vi "Get Camera Configuration.vi"(8 "error in (no error)":errorcluster, 11 "NI Vision Camera in":refnum<class "NI Vision Camera.lvclass">) -> (0 "error out":errorcluster, 2 "Configuration":T1, 3 "NI Vision Camera out":refnum<class "NI Vision Camera.lvclass">)   [LabVIEW 2014, in "NI Vision Camera.lvclass"]
uses:
  NI Vision Camera.lvclass
  Configuration.ctl
  NI Vision Camera.lvclass/NI Vision Camera.ctl
  <resource>/objmgr/imaqdx.rc
  Framework/Interfaces/Observable Actor/Observable Actor.lvclass
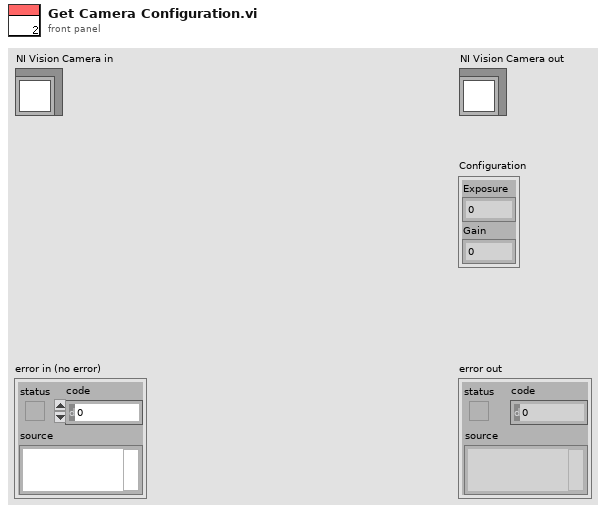
[diagram p1: front panel]
types:
  T1 = typedef "NI Vision Camera.lvclass/Configuration.ctl" = cluster{"Exposure":dbl, "Gain":dbl}
  T2 = typedef "IMAQdx.ctl" = refnum<k21>
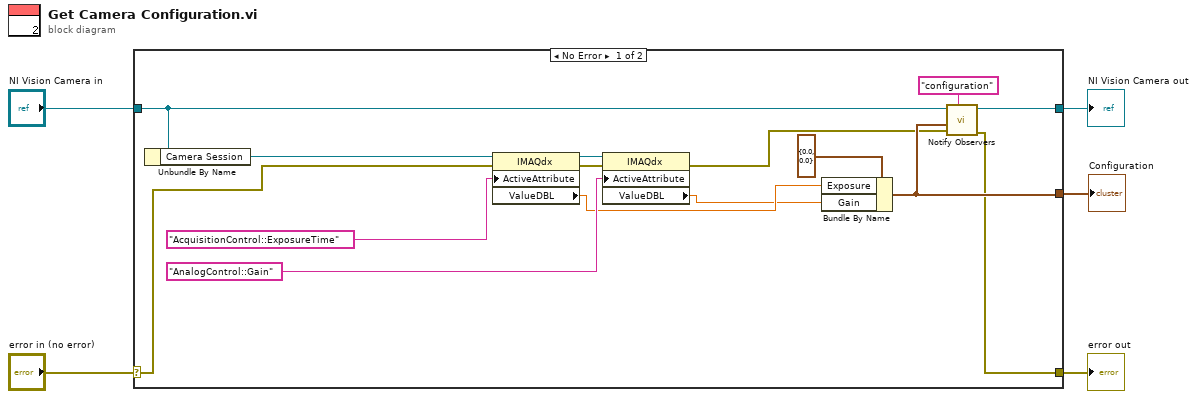
[diagram p0: block diagram]
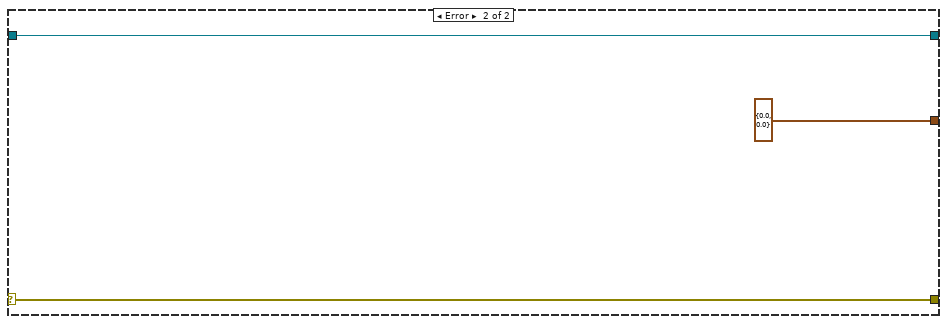
[diagram p2: hidden frame]
diagram:
  n1 = case shown="No Error" "error in (no error)" {
    selector: "error in (no error)" -> [w18 w23]
    tunnel: [w7 w23] -> w4
    tunnel: [w10 w22] -> w2
    tunnel: "NI Vision Camera in" -> [w11 w22]
    tunnel: [w9 T1 {"Exposure"=0.0, "Gain"=0.0} ("Configuration 2")] -> w1
    frame No Error {
      n2 = Unbundle By Name(w11) -> ("Camera Session"=w6:T2)
      n3 = property class="IMAQdx"(reference=w6, error in=w18, "ActiveAttribute"="AcquisitionControl::ExposureTime") -> (reference out=w20:T2, error out=w19:errorcluster, "ValueDBL"=w14:dbl)
      n4 = property class="IMAQdx"(reference=w20, error in=w19, "ActiveAttribute"="AnalogControl::Gain") -> (error out=w8:errorcluster, "ValueDBL"=w13:dbl)  [unwired: 1 out]
      n5 = Bundle By Name(cluster=T1 {"Exposure"=0.0, "Gain"=0.0} ("Configuration 2"), "Exposure"=w14, "Gain"=w13) -> (w9:T1)
      n6 = call "Notify Observers.vi"("name"="configuration", "error in (no error)"=w8, "value"=w9, "Observable Actor in"=w11) -> ("error out"=w7:errorcluster, "Observable Actor out"=w10:refnum<class "NI Vision Camera.lvclass">)  [unwired: 6 in]
    }
    frame Error {
    }
  }
  "error out" <- w4
  "NI Vision Camera out" <- w2
  "Configuration" <- w1
